vi "Untitled 2 (SubVI).vi"(11 "String in":string) -> (3 "String out":string)   [LabVIEW 2017]
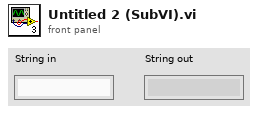
[diagram p1: front panel]
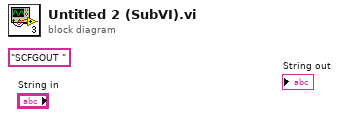
[diagram p0: block diagram]
diagram:
  w2 = "SCFGOUT "
